vi "file -- open-create folder.vi"(8 "folder name":string, 11 "base path":path) -> (3 "folder path out":path)   [LabVIEW 2015]
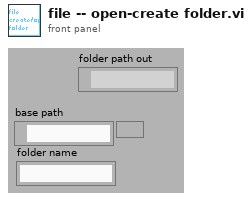
[diagram p1: front panel]
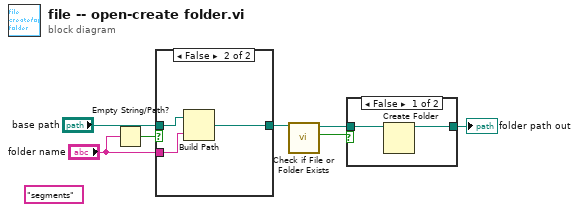
[diagram p0: block diagram]
diagram:
  (unwired) "segments" ("name or relative path")
  n1 = Empty String/Path?(string/path="folder name") -> (empty?=w7:bool)
  n2 = case shown="False" w7 {
    tunnel: "folder name" -> [_ w11]
    tunnel: "base path" -> [w8 w10]
    tunnel: [w8 w9] -> w4
    frame True {
    }
    frame False {
      n3 = Build Path(base path=w10, name or relative path=w11) -> (appended path=w9:path)
    }
  }
  n4 = call <vilib>:"Check if File or Folder Exists.vi"("path"=w4) -> ("file or folder exists?"=w2:bool, "dup path"=w3:path)  [unwired: 8 in, 1 out]
  n5 = case shown="False" w2 {
    tunnel: [w12 w14] -> w1
    tunnel: w3 -> [w13 w14]
    frame False {
      n6 = Create Folder(path (use dialog)=w13) -> (created path=w12:path)  [unwired: 2 in, 2 out]
    }
    frame True {
    }
  }
  "folder path out" <- w1
